vi "Actual Sample Mode.vi"(8 "error in (no error)":errorcluster {"code" format="%.0x"}, 11 "VISA Resource Name":refnum<visa-resource-name>) -> (0 "error out":errorcluster {"code" format="%.0x"}, 2 "Sample Mode":i32(ring) items=["Real Time", "Equivalent Time"], 3 "VISA Resource Name Out":refnum<visa-resource-name>)   [LabVIEW 2011, in "Agilent 546XX Series.lvlib"]
doc: "This VI returns the sample mode the oscilloscope is currently using."
uses:
  Agilent 546XX Series.lvlib
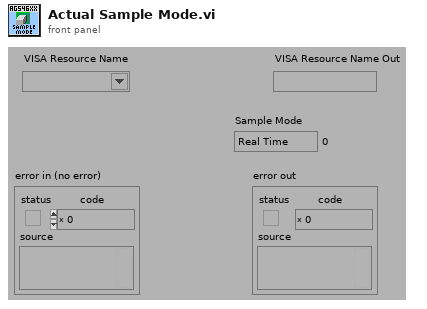
[diagram p1: front panel]
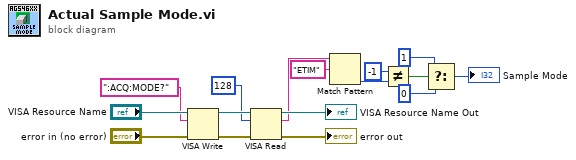
[diagram p0: block diagram]
diagram:
  n1 = VISA Write(VISA resource name="VISA Resource Name", write buffer=":ACQ:MODE?", error in (no error)="error in (no error)") -> (VISA resource name out=w16:refnum<visa-resource-name>, error out=w15:errorcluster)  [unwired: 1 out]
  n2 = VISA Read(VISA resource name=w16, byte count=u32 128, error in (no error)=w15) -> (VISA resource name out=→"VISA Resource Name Out":refnum<visa-resource-name>, read buffer=w8:string, error out=→"error out":errorcluster)  [unwired: 1 out]
  n3 = Match Pattern(string=w8, regular expression="ETIM") -> (offset past match=w6:i32)  [unwired: 1 in, 3 out]
  n4 = Not Equal?(x=-1, y=w6) -> (x != y?=w4:bool)
  n5 = Select(t=1, s=w4, f=0) -> (s? t:f=→"Sample Mode":i32)
